vi "Clear.vi"(8 "error in (no error)":errorcluster, 11 "Test Finder in":refnum<class "Test Finder.lvclass">) -> (0 "error out":errorcluster, 3 "Test Finder out":refnum<class "Test Finder.lvclass">)   [LabVIEW 2020, in "Test Finder.lvclass"]
uses:
  Test Finder.lvclass
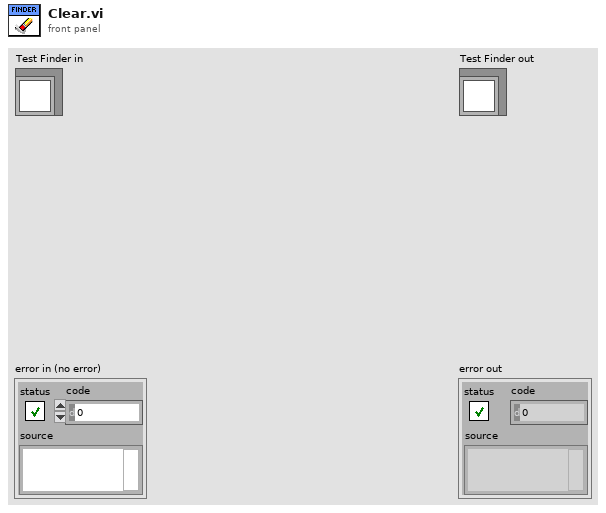
[diagram p1: front panel]
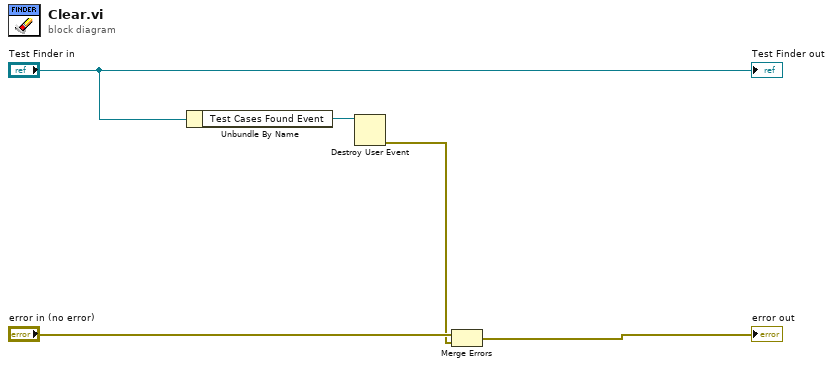
[diagram p0: block diagram]
diagram:
  n1 = Unbundle By Name("Test Finder in") -> ("Test Cases Found Event"=w3:refnum<user-event>)
  n2 = Destroy User Event(user event=w3) -> (error out=w1:errorcluster)  [unwired: 1 in]
  n3 = Merge Errors("error in (no error)", w1) -> (→"error out":errorcluster)
  "Test Finder out" <- "Test Finder in"
